vi "test Add Duplicate Alias.vi"(8 "error in (no error)":errorcluster, 11 "TestCase in":refnum<class "Routing and Faulting Aliases Unit Tests.lvclass">) -> (0 "error out":errorcluster, 3 "TestCase out":refnum<class "Routing and Faulting Aliases Unit Tests.lvclass">)   [LabVIEW 2020, in "Routing and Faulting Aliases Unit Tests.lvclass"]
uses:
  Routing and Faulting Aliases Unit Tests.lvclass
  Shared/Alias Mapping.ctl
  Shared/Alias Endpoint.ctl
  System Explorer/Alias.ctl
  System Explorer/Endpoint.ctl
  Routing and Faulting Aliases Unit Tests.lvclass/Routing and Faulting Aliases Unit Tests.ctl
  <vilib>/addons/_JKI Toolkits/VI Tester/TestCase.llb/TestCase.lvclass
  System Explorer/Routing and Faulting System Explorer.lvlib
  Scripting/Routing and Faulting Scripting.lvlib
  Shared/Routing and Faulting Shared.lvlib
  C:/Program Files (x86)/National Instruments/LabVIEW 2020/vi.lib/addons/_JKI Toolkits/VI Tester/TestCase.llb/TestCase.lvclass
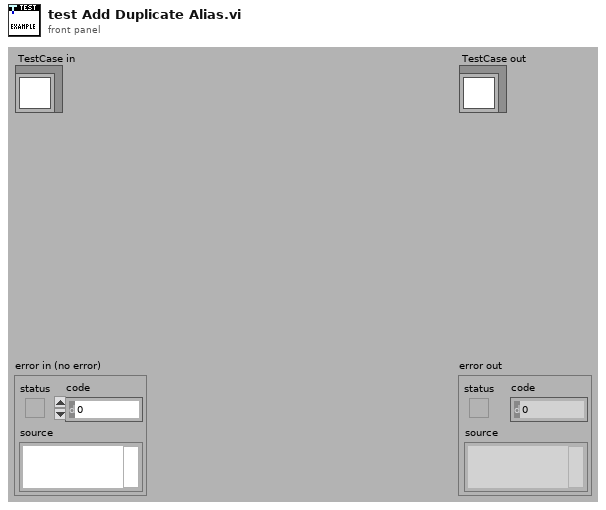
[diagram p1: front panel]
types:
  T1 = typedef "Routing and Faulting System Explorer.lvlib/Endpoint.ctl" = string
  T2 = typedef "Routing and Faulting Shared.lvlib/Alias Endpoint.ctl" = cluster{"Module Path":string, "Endpoint":string}
  T3 = typedef "Routing and Faulting System Explorer.lvlib/Alias.ctl" = cluster{"Endpoint":T1, "Alias":string, "Remove":bool}
  T4 = typedef "Routing and Faulting Shared.lvlib/Alias Mapping.ctl" = cluster{"Alias":string, "Endpoint":T2}
  T5 = typedef "Custom Device API.lvlib/Custom Device Item Ref.ctl" = u64
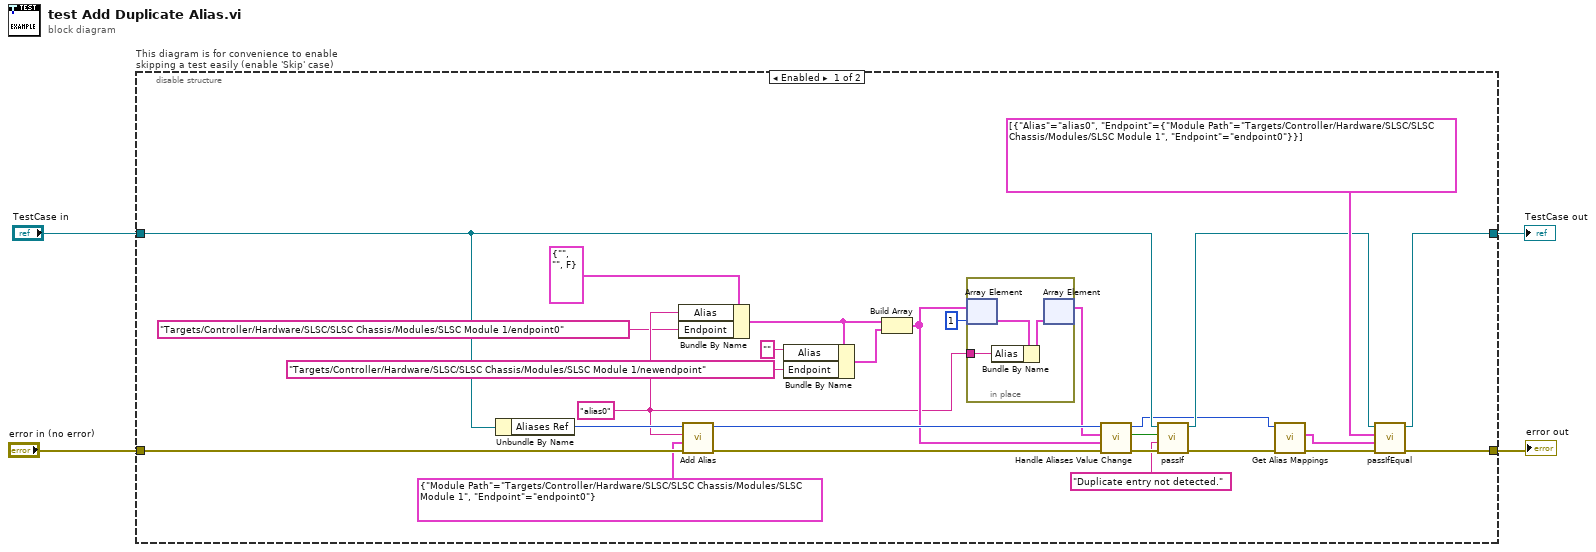
[diagram p0: block diagram]
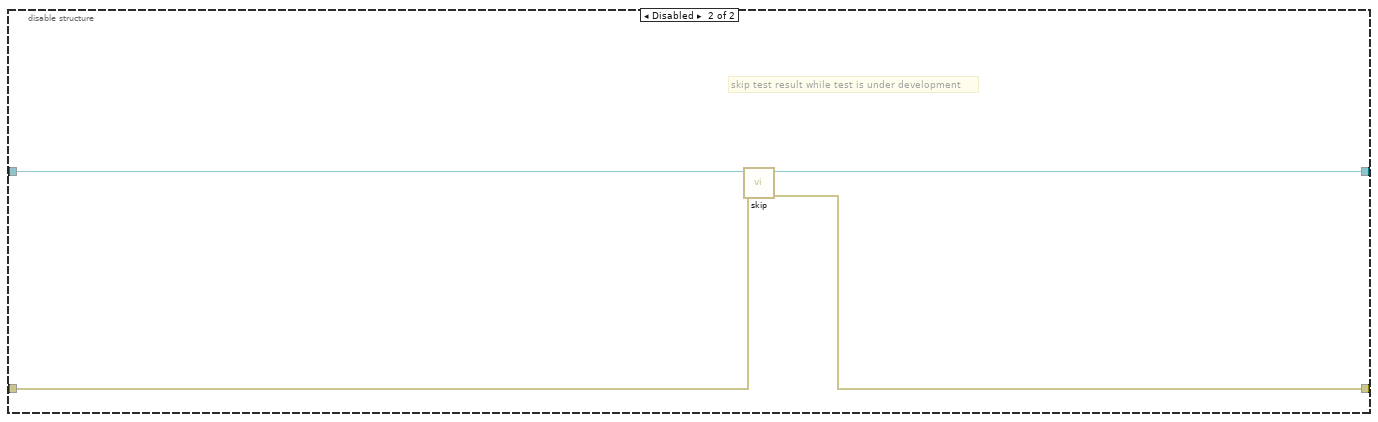
[diagram p2: hidden frame]
diagram:
  n1 = disable-structure "This diagram is for convenience to enable skipping a test easily (enable 'Skip' case)" shown="Enabled" {
    disable-tunnel: "TestCase in" -> [w12 w38]
    disable-tunnel: [w27 w36] -> w1
    disable-tunnel: [w30 w37] -> w3
    disable-tunnel: "error in (no error)" -> [w25 w35]
    frame Enabled {
      w15 = "alias0" ("Alias")
      n2 = Unbundle By Name(w12) -> ("Aliases Ref"=w26:T5)
      n3 = Bundle By Name(cluster=T3 {"Endpoint"="", "Alias"="", "Remove"=FALSE} ("Alias"), "Alias"=w15, "Endpoint"=T1 "Targets/Controller/Hardware/SLSC/SLSC Chassis/Modules/SLSC Module 1/endpoint0") -> (w19:T3)
      n4 = call "Add Alias.vi"("error in"=w25, "endpoint"=T2 {"Module Path"="Targets/Controller/Hardware/SLSC/SLSC Chassis/Modules/SLSC Module 1", "Endpoint"="endpoint0"} ("Endpoint"), "alias"=w15, "endpoint aliases in"=w26) -> ("error out"=w23:errorcluster, "endpoint aliases out"=w24:T5)  [unwired: 6 in]
      n5 = Bundle By Name(cluster=w19, "Alias"="", "Endpoint"=T1 "Targets/Controller/Hardware/SLSC/SLSC Chassis/Modules/SLSC Module 1/newendpoint") -> (w18:T3)
      n6 = Build Array(w19, w18) -> (w17:T3[])
      n7 = in-place {
        in-place-border: w15 -> [w32]
        n8 = in-place-array #1(w17, 1) -> (w34:T3)
        n9 = Bundle By Name(cluster=w34, "Alias"=w32) -> (w33:T3)
        n10 = in-place-array #1(w33) -> (w14:T3[])  [unwired: 1 out]
      }
      n11 = call "Handle Aliases Value Change.vi"("error in (no error)"=w23, "OldVal"=w17, "NewVal"=w14, "Aliases Ref in"=w24) -> ("error out"=w13:errorcluster, "Duplicate Entry"=w10:bool, "Aliases Ref out"=w7:T5)  [unwired: 4 in, 1 out]
      n12 = call-dynamic "passIf.vi"("error in (no error)"=w13, "message (\"\")"="Duplicate entry not detected." ("message (\"\")"), "pass"=w10, "TestCase in"=w12) -> ("error out"=w8:errorcluster, "TestCase out"=w11:refnum<class "Routing and Faulting Aliases Unit Tests.lvclass">)  [unwired: 6 in]
      n13 = call "Get Alias Mappings.vi"("error in"=w8, "endpoint aliases in"=w7) -> ("error out"=w31:errorcluster, "alias mappings"=w29:T4[])  [unwired: 7 in, 1 out]
      n14 = call-dynamic "passIfEqual.vi"("error in (no error)"=w31, "y"=w29, "x"=T4[] [{"Alias"="alias0", "Endpoint"={"Module Path"="Targets/Controller/Hardware/SLSC/SLSC Chassis/Modules/SLSC Module 1", "Endpoint"="endpoint0"}}] ("Alias Mappings"), "TestCase in"=w11) -> ("error out"=w30:errorcluster, "TestCase out"=w27:refnum<class "Routing and Faulting Aliases Unit Tests.lvclass">)  [unwired: 6 in]
    }
    frame Disabled {
      # "skip test result while test is under development"
      n15 = call <vilib>:"skip.vi"("error in (no error)"=w35, "TestCase in"=w38) -> ("error out"=w37:errorcluster, "TestCase out"=w36:refnum<class "Routing and Faulting Aliases Unit Tests.lvclass">)  [unwired: 8 in]
    }
  }
  "error out" <- w3
  "TestCase out" <- w1
